vi "Overlay Treatment Area.vi"(7 "Results":T1, 8 "Search":enum32{"Upper", "Lower"}(ring), 9 "Width":dbl, 10 "Location":dbl, 11 "Refnum in":T2) -> (3 "Refnum out":T2)   [LabVIEW 2015]
uses:
  <vilib>/vision/Image Controls.llb/IMAQ Image.ctl
  controls/Results.ctl
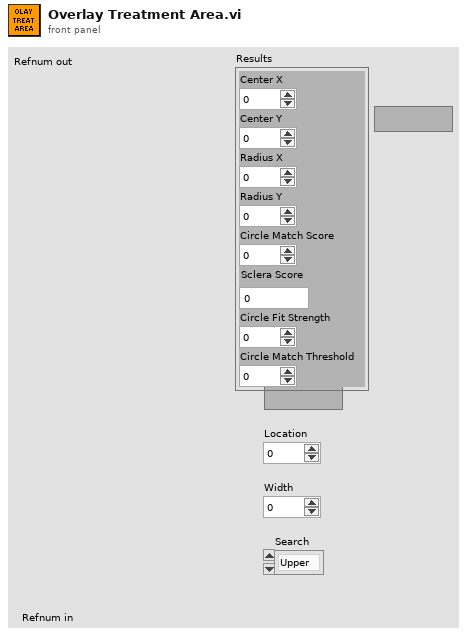
[diagram p1: front panel]
types:
  T1 = typedef "Results.ctl" = cluster{"Center X":i32, "Center Y":i32, "Radius X":i32, "Radius Y":i32, "Circle Match Score":i32, "Sclera Score":dbl, "Circle Fit Strength":i32, "Circle Match Threshold":i32}
  T2 = typedef "IMAQ Image.ctl" = refnum<image>
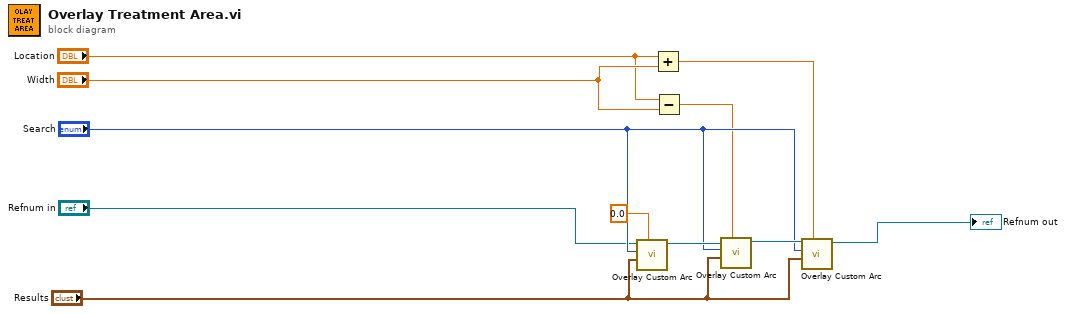
[diagram p0: block diagram]
diagram:
  n1 = call "Overlay Custom Arc.vi"("Offset"=0.0, "Results"="Results", "Search Area"="Search", "Refnum in"="Refnum in") -> ("Refnum out"=w9:T2)  [unwired: 7 in]
  n2 = Add(x="Location", y="Width") -> (x+y=w6:dbl)
  n3 = Subtract(x="Location", y="Width") -> (x-y=w5:dbl)
  n4 = call "Overlay Custom Arc.vi"("Offset"=w5, "Results"="Results", "Search Area"="Search", "Refnum in"=w9) -> ("Refnum out"=w10:T2)  [unwired: 7 in]
  n5 = call "Overlay Custom Arc.vi"("Offset"=w6, "Results"="Results", "Search Area"="Search", "Refnum in"=w10) -> ("Refnum out"=→"Refnum out":T2)  [unwired: 7 in]
